vi "_Main Async.vi"(10 "Server TCP Port":u16=4763, 11 "Server Address":string="127.0.0.1") -> ()   [LabVIEW 2020, in "LV Client.lvclass"]
uses:
  LV Client.lvclass
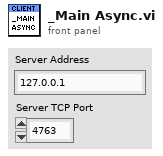
[diagram p1: front panel]
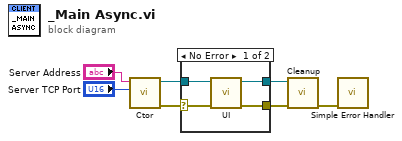
[diagram p0: block diagram]
diagram:
  n1 = call "Ctor.vi"("Server TCP Port"="Server TCP Port", "Server Address"="Server Address") -> ("error out"=w5:errorcluster, "LV Client out"=w4:refnum<class "LV Client.lvclass">)  [unwired: 8 in]
  n2 = case shown="No Error" w5 {
    selector: w5 -> [w10 w12]
    tunnel: w4 -> [w11 w13]
    tunnel: [w9 w13] -> w2
    tunnel: [w8 w12] -> w3
    frame No Error {
      n3 = call "UI.vi"("error in (no error)"=w10, "LV Client in"=w11) -> ("error out"=w8:errorcluster, "LV Client out"=w9:refnum<class "LV Client.lvclass">)  [unwired: 8 in]
    }
    frame Error {
    }
  }
  n4 = call "Cleanup.vi"("error in (no error)"=w3, "LV Client in"=w2) -> ("error out"=w1:errorcluster)  [unwired: 9 in]
  n5 = call <vilib>:"Simple Error Handler.vi"("error in (no error)"=w1) -> ()  [unwired: 4 in, 5 out]
